vi "Switch Close Refs.vi"(8 "error in (no error)":errorcluster, 11 "Switch Refs":refnum<k15>[](array[refnum])) -> (0 "error out":errorcluster)   [LabVIEW 2019]
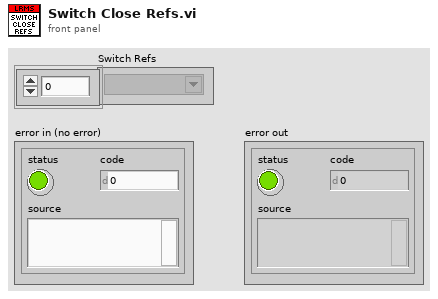
[diagram p1: front panel]
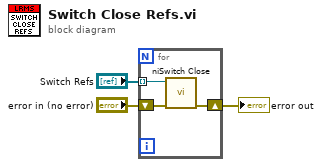
[diagram p0: block diagram]
diagram:
  n1 = for {
    shift-right: [w5] -> w1
    shift-left: "error in (no error)" -> [w6]
    tunnel: "Switch Refs" -> [w4] mode=indexing
    n2 = call <instrlib>:"niSwitch Close.vi"("error in (no error)"=w6, "instrument handle"=w4) -> ("error out"=w5:errorcluster)  [unwired: 9 in]
  }
  "error out" <- w1
